vi "Sample_SimpleContinuousRead.vi"() -> ()   [LabVIEW 2022 SP3, in "ADS_Library.lvlib"]
uses:
  ADS_Library.lvlib
  <userlib>/Beckhoff-LabVIEW-Interface/_DependsOn/Base/Read/Read Sync.vi
  <userlib>/Beckhoff-LabVIEW-Interface/_DependsOn/Base/TypeResolver/Get TypeResolver.vi
panel:
  out "Waveform Chart":dbl[](graph)
  in  "stop":bool
  out "Read status?":bool
  out "RDataArray":variant[](array[variant])
  out "RData":variant
  out "error out":errorcluster
  in  "error in":errorcluster
  in  "String":string="<PortInfo><Inputs><SymbolControlItems /></Inputs><Outputs><SymbolControlItems><SymbolControlItem GroupName=\"ADS Read\" GroupDescription=\"Parameters for ADS Read command\"><Parameters><Parameter Name=\"Name\">Term 9 (ELM3704-0000).PAI SamplesR32 1 Channel 1.Samples</Parameter><Parameter Name=\"SymbolName\">Term 9 (ELM3704-0000).PAI SamplesR32 1 Channel 1.Samples</Parameter><Parameter Name=\"SymbolType\">Samples_9BD8E00D</Parameter><Parameter Name=\"SymbolGuid\"></Parameter><Parameter Name=\"AmsNetId\">192.168.80.50.1.1</Parameter><Parameter Name=\"Port\">27906</Parameter><Parameter Name=\"IndexGroup\">#x0</Parameter><Parameter Name=\"IndexOffset\">#x0</Parameter><Parameter Name=\"BitSize\">32</Parameter><Parameter Name=\"CycleTime [ms]\">10</Parameter><Parameter Name=\"Transmode\">3</Parameter><Parameter Name=\"Timeout [ms]\">1000</Parameter><Parameter Name=\"TCBufferSize [Samples]\">10</Parameter><Parameter Name=\"LVBufferSize [Samples]\">50</Parameter><Parameter Name=\"Expected min delay [ms]\">500</Parameter></Parameters></SymbolControlItem></SymbolControlItems></Outputs></PortInfo>"
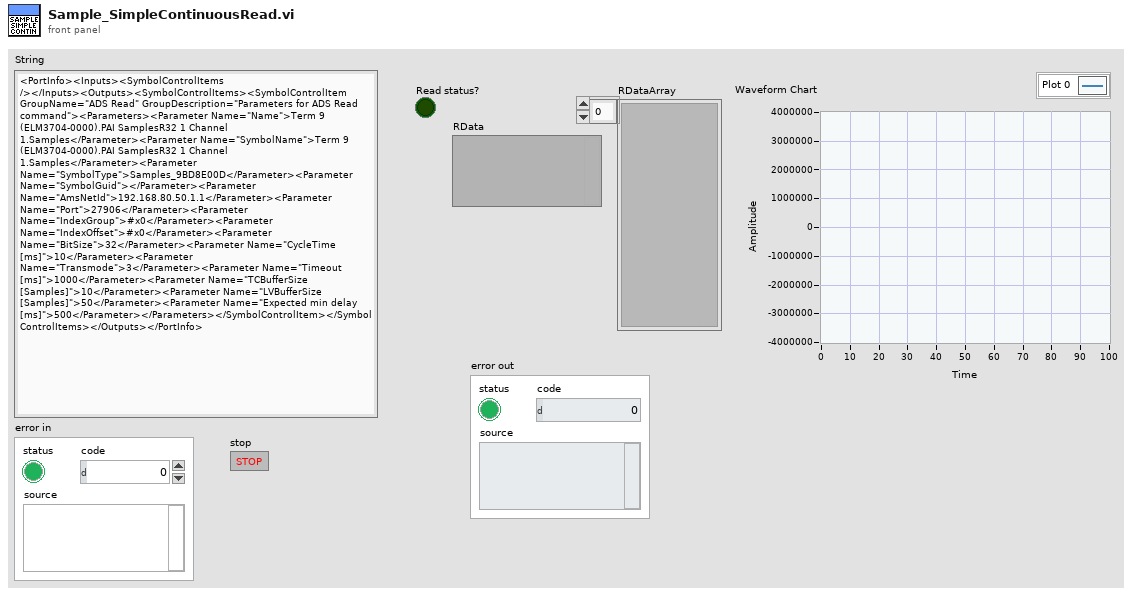
[diagram p1: front panel]
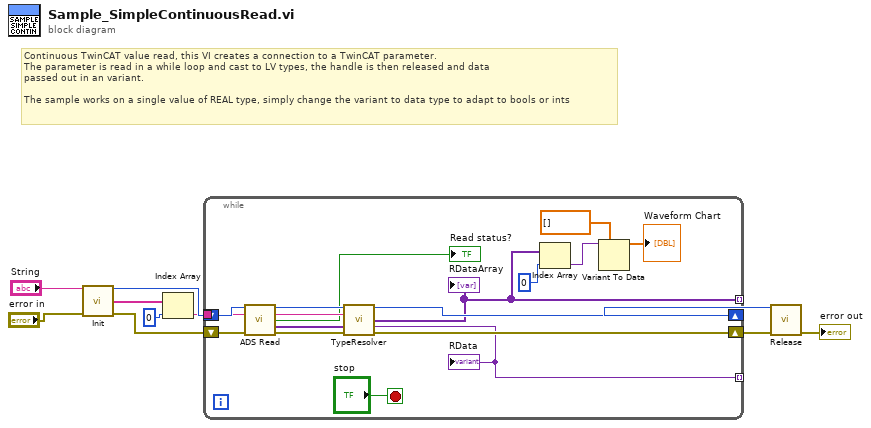
[diagram p0: block diagram]
diagram:
  # "Continuous TwinCAT value read, this VI creates a connection to a TwinCAT parameter.\nThe parameter is read in a while loop and cast to LV types, the handle is then released and data \npassed out in an variant. \n\nThe sample works on a single value of REAL type, simply change the variant to data type to adapt to bools or ints"
  n1 = call <userlib>:"Init.vi"("XMLDescription"="String", "error in (no error)"="error in") -> ("Handle"=w8:u32, "ReadGrpSymbols"=w7:string[], "error out"=w9:errorcluster)  [unwired: 9 in, 2 out]
  n2 = Index Array(array=w7, index=0) -> (element=w5:string)
  n3 = while {
    tunnel: w5 -> [w25]
    shift-right: [w20] -> w4
    shift-left: w9 -> [w27]
    shift-right: [w19] -> w3
    shift-left: w8 -> [w26]
    tunnel: [w13] -> _ mode=indexing
    tunnel: [w16] -> _ mode=indexing
    stop <- "stop" stop-if-true
    n4 = call-poly <userlib>:"ADS Read.vi"("Handle"=w26, "SymbolName"=w25, "error in (no error)"=w27) -> ("Handle"=w24:u32, "SymbolName"=w23:string, "Read status?"=→"Read status?":bool, "Ads Read Data"=w22:variant[], "error out"=w21:errorcluster)  [unwired: 8 in]
    n5 = call-poly <userlib>:"TypeResolver.vi"("Handle"=w24, "SymbolName"=w23, "ADSRData"=w22, "error in"=w21) -> ("Handle"=w19:u32, "RDataArray"=w13:variant[], "RData"=w16:variant, "error out"=w20:errorcluster)  [unwired: 8 in]
    "RDataArray" <- w13
    "RData" <- w16
    n6 = Index Array(array=w13, index=0) -> (element=w11:variant)
    n7 = Variant To Data(type=dbl[] [], Variant=w11) -> (data=→"Waveform Chart":dbl[])  [unwired: 1 in, 1 out]
  }
  n8 = call <userlib>:"Release.vi"("Handle"=w3, "error in (no error)"=w4) -> ("error out"=→"error out":errorcluster)  [unwired: 13 in]
